vi "setOutputState.vi"(7 "chn":string, 8 "error in (no error)":errorcluster, 10 "state":bool, 11 "PsuNiPxi in":refnum<class "PsuNi.lvclass">) -> (0 "error out":errorcluster, 3 "PsuNiPxi out":refnum<class "PsuNi.lvclass">)   [LabVIEW 2023, in "PsuNi.lvclass"]
doc: "<b>Author:</b> Wolfgang\n<b>Description:</b> set output state of power supply by channel, true = on; false = off"
uses:
  PsuNi.lvclass
  PsuNi.lvclass/PsuNi.ctl
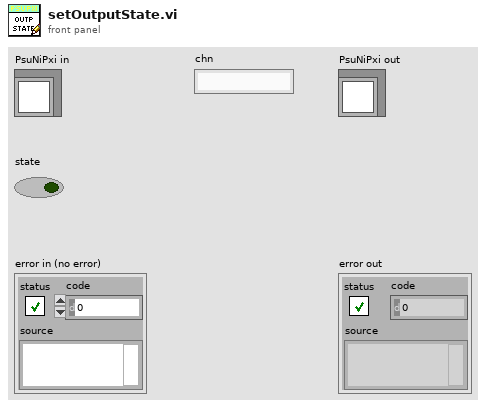
[diagram p1: front panel]
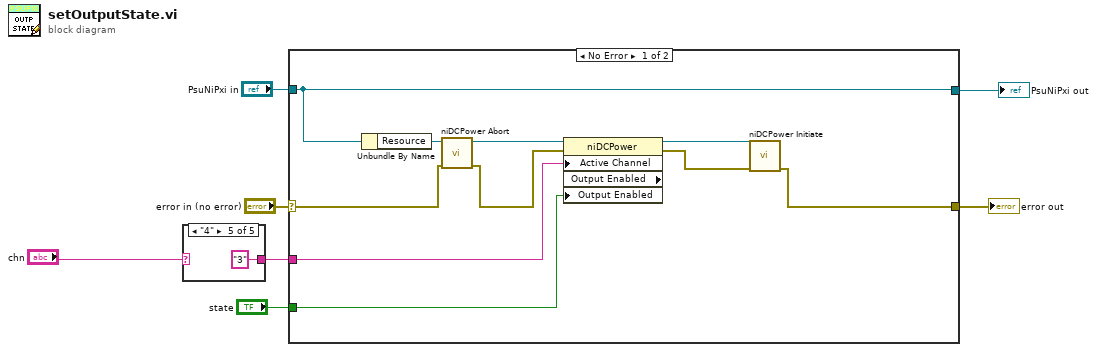
[diagram p0: block diagram]
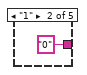
[diagram p3: hidden frame]
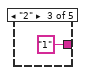
[diagram p4: hidden frame]
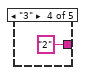
[diagram p5: hidden frame]
diagram:
  n1 = case shown="\"4\"" "chn" {
    selector: "chn" -> [w8 _ _ _ _]
    tunnel: [w8 "0" "1" "2" "3"] -> w2
    frame "False", Default {
    }
    frame "1" {
    }
    frame "2" {
    }
    frame "3" {
    }
    frame "4" {
    }
  }
  n2 = case shown="No Error" "error in (no error)" {
    selector: "error in (no error)" -> [w14 w23]
    tunnel: [w17 w23] -> w7
    tunnel: [w22 w24] -> w6
    tunnel: "PsuNiPxi in" -> [w22 w24]
    tunnel: w2 -> [w19 _]
    tunnel: "state" -> [w16 _]
    frame No Error {
      n3 = Unbundle By Name(w22) -> ("Resource"=w21:refnum<k15>)
      n4 = call <instrlib>:"niDCPower Abort.vi"("error in (no error)"=w14, "instrument handle"=w21) -> ("error out"=w13:errorcluster, "instrument handle out"=w15:refnum<k15>)  [unwired: 8 in]
      n5 = property class="niDCPower" props=["Active Channel", "Output Enabled", "Output Enabled"](reference=w15, error in=w13, "Active Channel"=w19, "Output Enabled"=w16) -> (reference out=w20:refnum<k15>, error out=w18:errorcluster)  [unwired: 1 out]
      n6 = call <instrlib>:"niDCPower Initiate.vi"("error in (no error)"=w18, "instrument handle"=w20) -> ("error out"=w17:errorcluster)  [unwired: 8 in, 1 out]
    }
    frame Error {
    }
  }
  "error out" <- w7
  "PsuNiPxi out" <- w6
